vi "图像数据归一化.vi"(1 "N-1":i32, 2 "Data":dbl[][](array[numeric])) -> (0 "Normlized":dbl[][](array[numeric]))   [LabVIEW 2018]
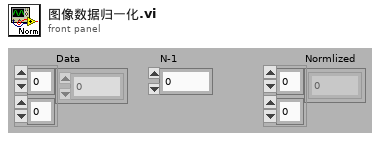
[diagram p1: front panel]
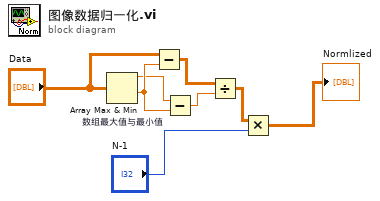
[diagram p0: block diagram]
diagram:
  n1 = Array Max & Min "数组最大值与最小值"(array="Data") -> (max value=w2:dbl, min value=w3:dbl)  [unwired: 2 out]
  n2 = Subtract(x="Data", y=w3) -> (x-y=w4:dbl[][])
  n3 = Subtract(x=w2, y=w3) -> (x-y=w5:dbl)
  n4 = Divide(x=w4, y=w5) -> (x/y=w7:dbl[][])
  n5 = Multiply(x=w7, y="N-1") -> (x*y=→"Normlized":dbl[][])
